vi "aal_DZT (complex input).vi"(0 "x":cdb[](array[numeric]), 1 "M":i32, 2 "index":i32, 3 "out_len":i32, 4 "fft_len":i32) -> (5 "Y":cdb[](array[numeric]), 6 "error":i32)   [LabVIEW 2010, in "NI_AALPro.lvlib"]
doc: "This function returns portion of single side band FFT of a real input signal.\n\nInputs:\n\n M : zoom in factor\n x : real input signal, with length of x_len\n index : initial index of the signal side band FFT where the \"zoom-in\" FFT starts.\n\noutputs:\n Y : output of the \"zoom in\" FFT with length of x_len/M/2. .\n\nSome restrictions applied on the input parameters:\n1. Signal length (x_len) must be mutiple of zoom in factor M.\n2. index >= 0, and (index+x_len/M/2)<x_len/2."
uses:
  NI_AALPro.lvlib
  lvanlys.dll
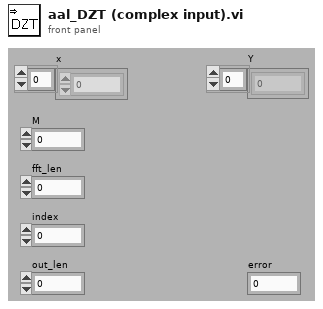
[diagram p1: front panel]
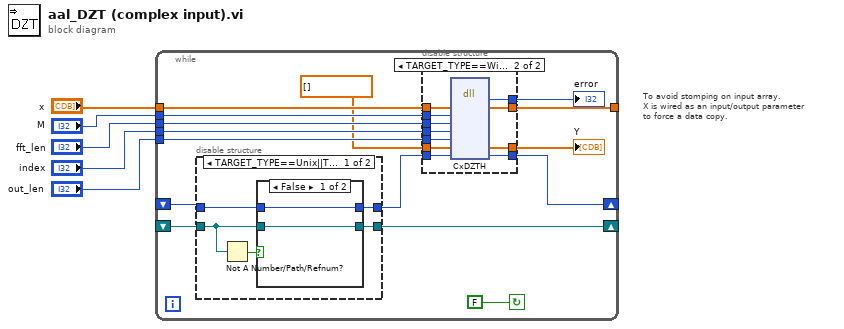
[diagram p0: block diagram]
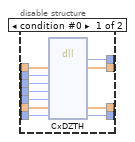
[diagram p2: hidden frame]
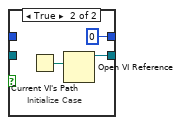
[diagram p3: hidden frame]
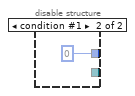
[diagram p4: hidden frame]
diagram:
  # "To avoid stomping on input array. \nX is wired as an input/output parameter \nto force a data copy."
  n1 = while {
    shift-left: _ -> [w12]
    shift-right: [w14] -> _
    tunnel: "fft_len" -> [w15]
    tunnel: "index" -> [w16]
    tunnel: "out_len" -> [w17]
    tunnel: "M" -> [w18]
    tunnel: "x" -> [w20]
    shift-right: [w11] -> _
    shift-left: _ -> [w9]
    tunnel: [w8] -> _
    stop <- FALSE continue-if-true
    n2 = disable-structure shown="TARGET_TYPE==Unix||TARGET_TYPE==Mac||TARGET_TYPE==RT||TARGET_TYPE==Windows, default" {
      disable-tunnel: [w46 _] -> w11
      disable-tunnel: [w45 0 ("t")] -> w10
      disable-tunnel: w12 -> [w44 _]
      disable-tunnel: w9 -> [w43 _]
      frame condition #0 (active) {
        n3 = Not A Number/Path/Refnum?(number/path/refnum=w43) -> (NaN/Path/Refnum?=w47:bool)
        n4 = case shown="False" w47 {
          tunnel: [w48 w51] -> w46
          tunnel: [w49 0 ("error")] -> w45
          tunnel: w44 -> [w49 _]
          tunnel: w43 -> [w48 _]
          frame False {
          }
          frame True {
            # "Initialize Case"
            n5 = Current VI's Path() -> (path=w52:path)
            n6 = Open VI Reference(vi path=w52) -> (vi reference=w51:refnum<vi>)  [unwired: 5 in, 1 out]
          }
        }
      }
      frame condition #1 {
      }
    }
    n7 = disable-structure shown="TARGET_TYPE==Windows||TARGET_TYPE==Mac||TARGET_TYPE==Unix" {
      disable-tunnel: w20 -> [w31 w42]
      disable-tunnel: [w30 w41] -> w19
      disable-tunnel: w18 -> [w29 w40]
      disable-tunnel: w17 -> [w28 w39]
      disable-tunnel: w16 -> [w27 w38]
      disable-tunnel: w15 -> [w26 w37]
      disable-tunnel: [w25 w36] -> w14
      disable-tunnel: w10 -> [w24 w35]
      disable-tunnel: [w23 w34] -> w7
      disable-tunnel: [w22 w33] -> w8
      disable-tunnel: cdb[] [] ("Y") -> [w21 w32]
      frame condition #0 {
        n8 = dll-call lib="C:/Program Files/National Instruments/LabVIEW 2010/resource/lvanlys.dll" fn="CxDZTH"("x"=w31, "M"=w29, "fft_len"=w26, "index"=w27, "out_len"=w28, w21, "tbl"=w24) -> (w30:i32, "x"=w22:cdb[], w23:cdb[], "tbl"=w25:i32)  [unwired: 7 in, 2 out]
      }
      frame condition #1 (active) {
        n9 = dll-call lib="C:/Program Files/National Instruments/LabVIEW 2010/resource/lvanlys.dll" fn="CxDZTH"("x"=w42, "M"=w40, "fft_len"=w37, "index"=w38, "out_len"=w39, "y"=w32, "tbl"=w35) -> ("return type"=w41:i32, "x"=w33:cdb[], "y"=w34:cdb[], "tbl"=w36:i64)  [unwired: 7 in, 2 out]
      }
    }
    "error" <- w19
    "Y" <- w7
  }
